vi "Control Stop.vi"(1 "error":i32=-1600) -> ()   [LabVIEW 2017, in "NI_AdvCtrl_continuous linear.lvlib"]
doc: "LabVIEW no longer supports this VI. You can obtain similar functionality by installing the LabVIEW Simulation Module."
uses:
  <vilib>/addons/control/advanced/NI_AdvCtrl_continuous linear.lvlib
  <vilib>/addons/control/advanced/continuous linear.llb/global autotest.vi
panel:
  in  "error text":string[](array[string])=["upper bound<lower bound (Limited Integrator)", "numerator/denominator inconsistency", "highest coefficient of a polynomial close to 0", "ill-conditioned MIMO system", "failure in discrete filter specification", "quantization interval negative", "switch on/off problem (Relay)", "upper limit<lower limit (Saturation)", "size of input points and initial conditions are not the same (Integrator)", "size of input points and initial conditions are not the same (Limited Integrator)", "size of input points and initial conditions are not the same (Derivative)", "size of input points and transfer functions are not the same (Transfer Function)", "size of input points and zeros-poles-gains are not the same (Zero Pole)", "size of input points and initial conditions are not the same (Discrete Integrator)", "size of input points, initial conditions, and bounds are not the same (Discrete Limited Integrator)", "size of input points and filter coefficients are not the same (Discrete Filter)", "size of input points and transfer functions are not the same (Discrete Transfer Function)", "size of input points and zeros-poles-gains are not the same (Discrete Zero Pole)", "size of input points and initial conditions are not the same (Unit Delay)", "size of input points and initial conditions are not the same (Memory)", "size of input points and initial conditions are not the same (Initial Condition)", "size of input points and initial conditions are not the same (State Space)", "size of input points and initial conditions are not the same (Discrete State Space)"]
  in  "error codes":i32[](array[numeric])=[-1600, -1601, -1602, -1603, -1604, -1605, -1606, -1607, -1608, -1609, -1610, -1611, -1612, -1613, -1614, -1615, -1616, -1617, -1618, -1619, -1620, -1621, -1622]
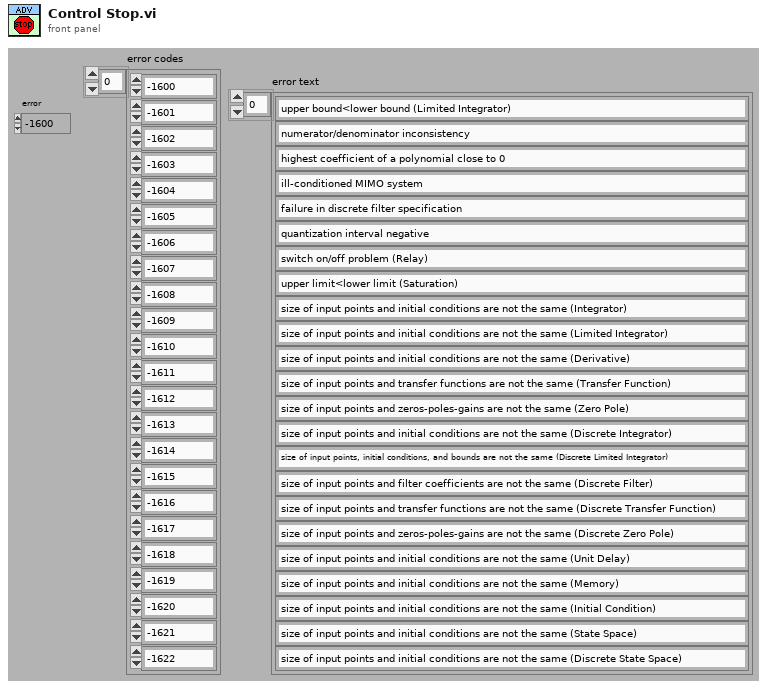
[diagram p1: front panel]
types:
  T1 = cluster{"auto test":bool, "error":i32, "spreadsheet string":string}
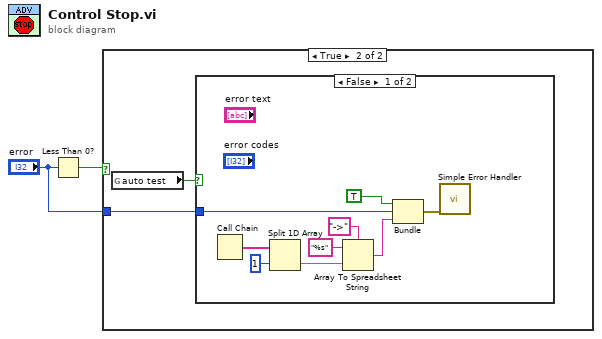
[diagram p0: block diagram]
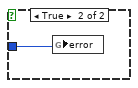
[diagram p3: hidden frame]
diagram:
  n1 = Less Than 0?(x="error") -> (x < 0?=w2:bool)
  n2 = case shown="True" w2 {
    tunnel: "error" -> [_ w4]
    frame False {
    }
    frame True {
      n3 = global read "global autotest.vi" "auto test"() -> (w3:bool)
      n4 = case shown="False" w3 {
        tunnel: w4 -> [w13 w14]
        frame False {
          n5 = Call Chain() -> (call chain=w7:string[])
          n6 = Split 1D Array(array=w7, index=1) -> (second subarray=w5:string[])  [unwired: 1 out]
          n7 = Array To Spreadsheet String(delimiter (Tab)="->", array=w5, 3:"%s" ("format string")) -> (spreadsheet string=w8:string)
          n8 = Bundle("auto test"=TRUE, "error"=w13, "spreadsheet string"=w8) -> (w11:T1)  [unwired: 1 out]
          n9 = call <vilib>:"Simple Error Handler.vi"("error in (no error)"=w11) -> ()  [unwired: 1 in, 8 out]
        }
        frame True {
          n10 = global write "global autotest.vi" "error"(w14) -> ()
        }
      }
    }
  }
